vi "PeekQueueMain.vi"(0 "object in":refnum<class "Application.lvclass">=refnum, 5 "error in (no error)":errorcluster) -> (14 "object out":refnum<class "Application.lvclass">, 16 "Message":string, 17 "Message Data":variant=variant(errorcluster {"status"=TRUE, "code"=1, "source"="MainTemplate.vi<ERR>\nThe invalid message string \"\" was received in the Message Handling Loop.\n\n\n<b>Complete call chain:</b>\r\n     MainTemplate.vi"}), 19 "error out":errorcluster)   [LabVIEW 2021, in "Application.lvclass"]
uses:
  Application.lvclass
  Hamamatsu_class/Hamamatsu.lvclass
  AD2_SDK_class/AD2_SDK.lvclass
  Valve_class/Valve.lvclass
  Ismatec_class/Ismatec.lvclass
  ExperimentSeries_class/ExperimentSeries.lvclass
  CetoniPump_class/CetoniPump.lvclass
  Prior_Zmotor_class/Prior_Zmotor.lvclass
  ExperimentSeries2_class/ExperimentSeries2.lvclass
  Application.lvclass/Application.ctl
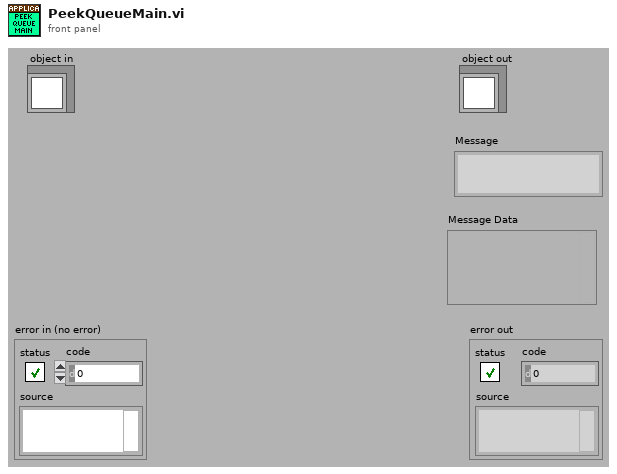
[diagram p1: front panel]
types:
  T1 = cluster{"Message":string, "Message Data":variant}
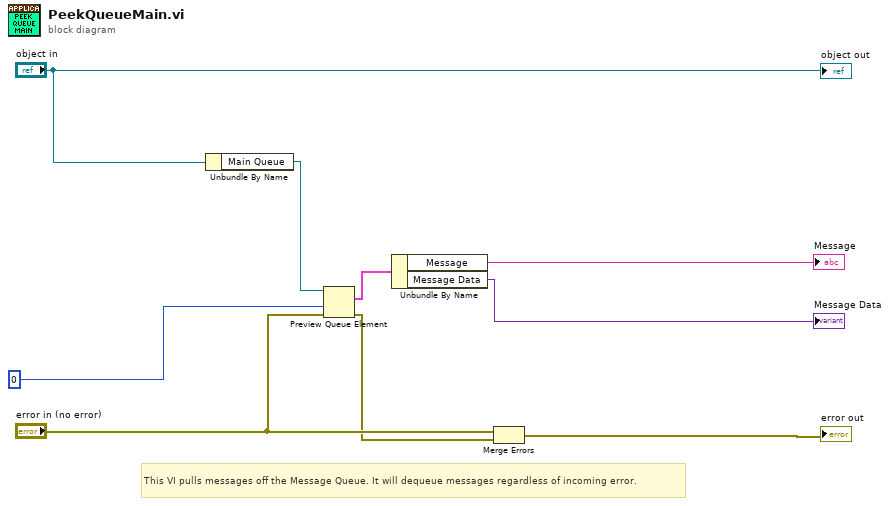
[diagram p0: block diagram]
diagram:
  # "This VI pulls messages off the Message Queue. It will dequeue messages regardless of incoming error."
  n1 = Unbundle By Name("object in") -> ("Main Queue"=w5:refnum<queue>)
  n2 = Preview Queue Element(queue=w5, timeout in ms (-1)=0, error in (no error)="error in (no error)") -> (element=w4:T1, error out=w1:errorcluster)  [unwired: 2 out]
  n3 = Unbundle By Name(w4) -> ("Message"=→"Message":string, "Message Data"=→"Message Data":variant)
  n4 = Merge Errors("error in (no error)", w1) -> (→"error out":errorcluster)
  "object out" <- "object in"
